vi "LED Configure.vi"(9 "LED On":bool, 10 "refnum name":string, 11 "LEDChannel":T1) -> ()   [LabVIEW 2019]
uses:
  <vilib>/Rock Robotics/WPI/ThirdParty/Phoenix-LabVIEW/CANifier/CTRE_CANifier_LEDChannel.ctl
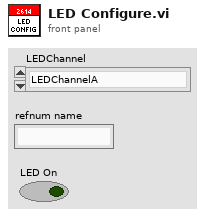
[diagram p1: front panel]
types:
  T1 = typedef "CTRE_CANifier_LEDChannel.ctl" = enum32{"LEDChannelA", "LEDChannelB", "LEDChannelC"}
  T2 = typedef "CTRE_CANifier_DeviceRef.ctl" = cluster{"DeviceStatus":errorcluster, "Device Number":u8, "Handle":u64, "UsageFrame":u32, "Library Path":path}
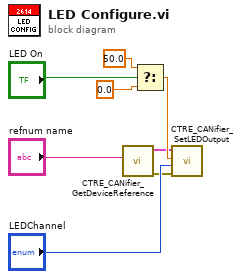
[diagram p0: block diagram]
diagram:
  n1 = call <vilib>:"CTRE_CANifier_GetDeviceReference.vi"("refnum name"="refnum name") -> ("error out"=w3:errorcluster, "CANifierDevRef"=w2:T2)  [unwired: 9 in]
  n2 = Select(t=50.0, s="LED On", f=0.0) -> (s? t:f=w8:dbl)
  n3 = call <vilib>:"CTRE_CANifier_SetLEDOutput.vi"("error in"=w3, "LEDChannel"="LEDChannel", "Percent Output"=w8, "CANifierDevRef"=w2) -> ()  [unwired: 6 in, 2 out]
